vi "Exactly Tolerant Inputs.vi"(7 "Expected Number of Calls":u32, 8 "error in (no error)":errorcluster, 10 "Tolerance":dbl, 11 "Mock in":refnum<class "LMock Mock.lvclass">) -> (0 "error out":errorcluster, 3 "Mock out":refnum<class "LMock Mock.lvclass">)   [LabVIEW 2020, in "Exactly.lvlib"]
uses:
  Exactly.lvlib
  Framework/Mock/LMock Mock.lvclass
  Comparators/Tolerant Numeric Input Comparator/Tolerant Numeric Input Comparator.lvclass/Tolerant Numeric Input Comparator.ctl
  Comparators/Tolerant Numeric Input Comparator/Tolerant Numeric Input Comparator.lvclass
  C:/git/astemes-lmock/source/Core/Comparator/Comparator.lvclass
  Exactly.lvclass
  C:/git/astemes-lmock/source/Core/Expectation/Expectation.lvclass
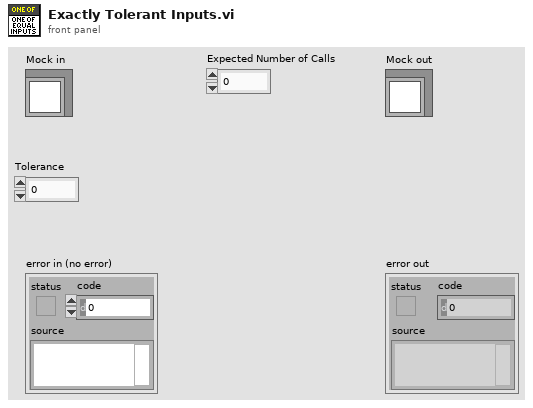
[diagram p1: front panel]
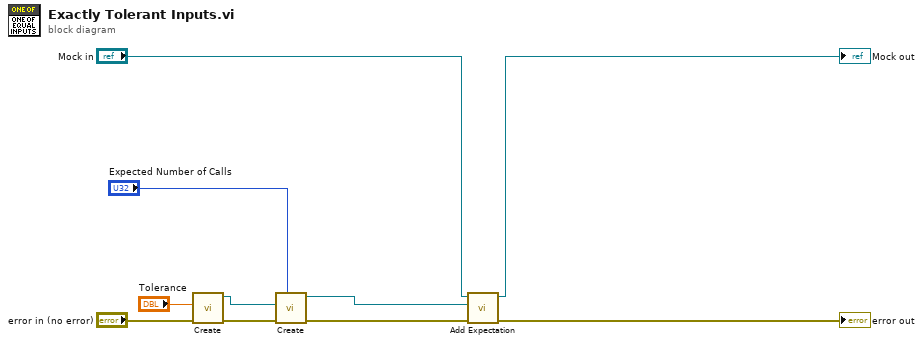
[diagram p0: block diagram]
diagram:
  n1 = call "Create.vi"("error in (no error)"="error in (no error)", "Tolerance"="Tolerance") -> ("error out"=w3:errorcluster, "Tolerant Numeric Comparator Out"=w5:refnum<class "Tolerant Numeric Input Comparator.lvclass">)  [unwired: 8 in]
  n2 = call "Create.vi"("Expected Number of Calls"="Expected Number of Calls", "error in (no error)"=w3, "Comparator"=w5) -> ("error out"=w7:errorcluster, "Exactly Out"=w6:refnum<class "Exactly.lvclass">)  [unwired: 7 in]
  n3 = call-dynamic "Add Expectation.vi"("error in (no error)"=w7, "Expectations"=w6, "Mock in"="Mock in") -> ("error out"=→"error out":errorcluster, "Mock out"=→"Mock out":refnum<class "LMock Mock.lvclass">)  [unwired: 7 in]
